vi "Get subnet.vi"() -> (14 "Subnet":string[](array[string]))   [LabVIEW 2026]
doc: "Calls system specific operating system function and returns subnet broadcast addresses of all installed network cards. Supports Windows (default case, calls IPCONFIG), Unix (calls IFCONFIG) and Mac.OS (calls IFCONFIG)."
panel:
  out "IP address":string[](array[string])
  out "Subnet mask":string[](array[string])
  out "Sum":i32[][](array[numeric])
  out "IPCONFIG Output":string
  # "Calls IPCONFIG and returns subnet broadcast addresses of all installed network cards."
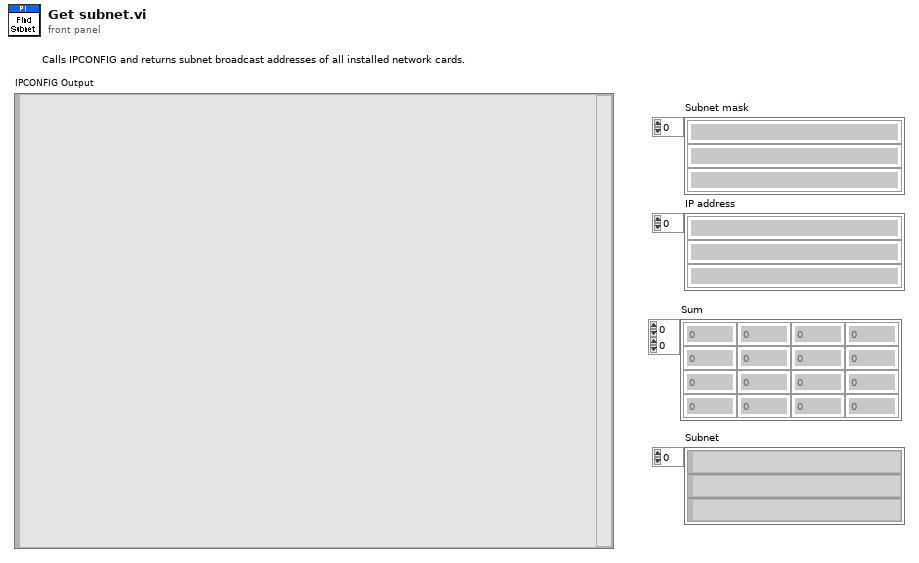
[diagram p1: front panel]
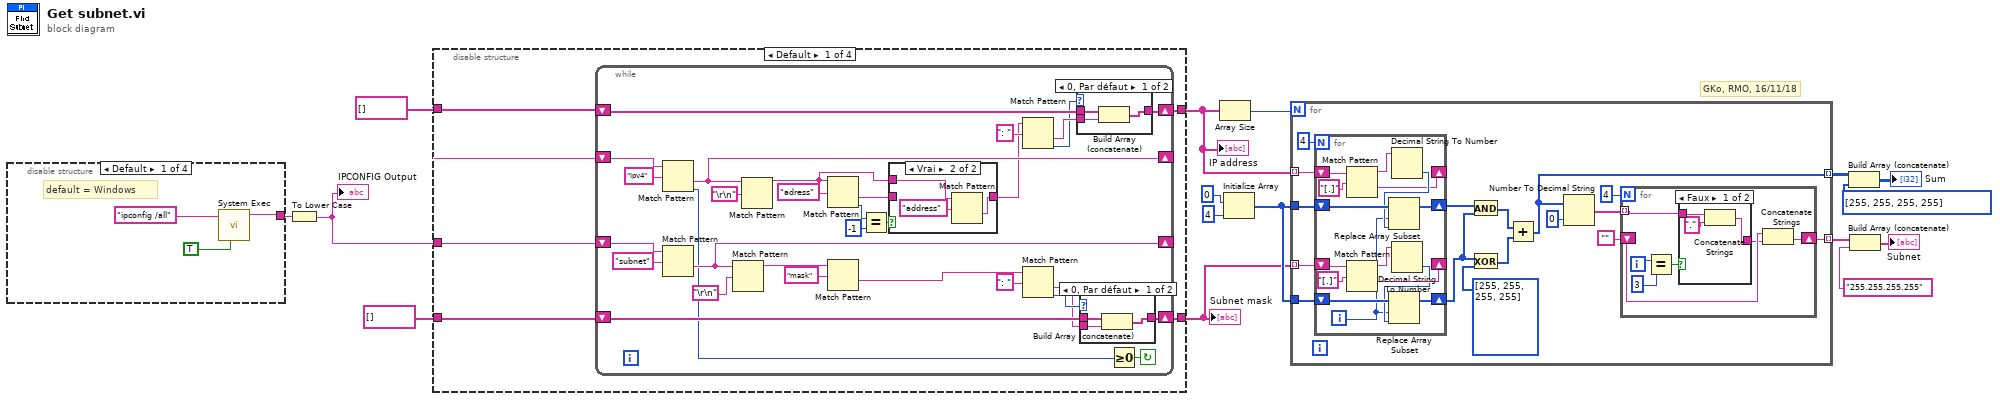
[diagram p0: block diagram]
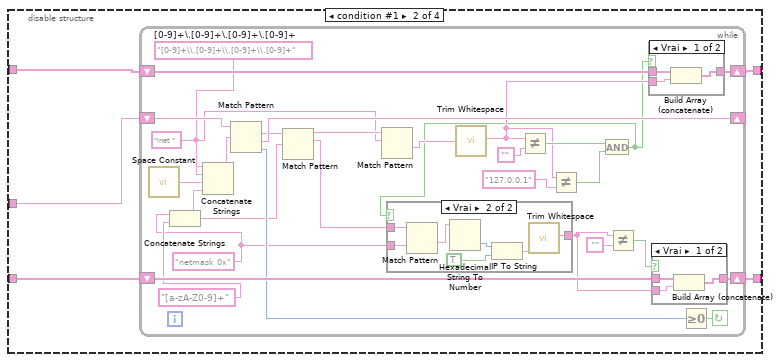
[diagram p5: hidden frame]
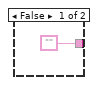
[diagram p6: hidden frame]
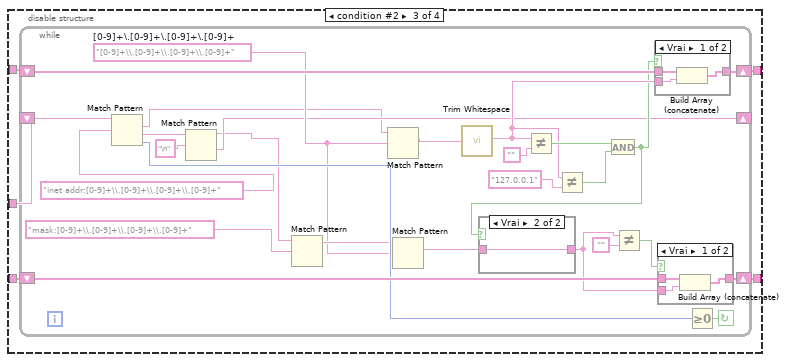
[diagram p9: hidden frame]
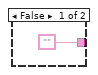
[diagram p10: hidden frame]
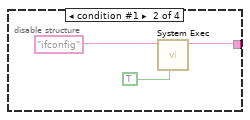
[diagram p14: hidden frame]
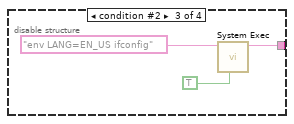
[diagram p15: hidden frame]
diagram:
  # "GKo, RMO, 16/11/18"
  n1 = disable-structure shown="Default" {
    disable-tunnel: [w17 w20 w23 _] -> w1
    frame condition #0 (active) {
      # "default = Windows"
      n2 = call <vilib>:"System Exec.vi"("run minimized? (F)"=TRUE, "command line"="ipconfig /all") -> ("standard output"=w17:string)  [unwired: 4 in, 5 out]
    }
    frame condition #1 {
      n3 = call <vilib>:"System Exec.vi"("run minimized? (F)"=TRUE, "command line"="ifconfig") -> ("standard output"=w20:string)  [unwired: 4 in, 5 out]
    }
    frame condition #2 {
      n4 = call <vilib>:"System Exec.vi"("run minimized? (F)"=TRUE, "command line"="env LANG=EN_US ifconfig") -> ("standard output"=w23:string)  [unwired: 4 in, 5 out]
    }
    frame condition #3 {
      # "No broadcasts on RT systems"
    }
  }
  n5 = To Lower Case(string=w1) -> (all lower case string=w15:string)
  "IPCONFIG Output" <- w15
  n6 = disable-structure shown="Default" {
    disable-tunnel: string[] [] -> [w30 w75 w125 w164]
    disable-tunnel: w15 -> [w29 w76 w124 _]
    disable-tunnel: string[] [] -> [w28 w77 w126 w165]
    disable-tunnel: [w27 w73 w122 w164] -> w9
    disable-tunnel: [w26 w74 w123 w165] -> w8
    frame condition #0 (active) {
      n7 = while {
        shift-right: [w55] -> _
        shift-left: w29 -> [w60]
        shift-right: [w52] -> w27
        shift-left: w30 -> [w53]
        shift-right: [w37] -> _
        shift-left: w29 -> [w43]
        shift-right: [w40] -> w26
        shift-left: w28 -> [w41]
        stop <- w56 continue-if-true
        n8 = Match Pattern(string=w43, regular expression="ipv4") -> (after substring=w37:string, offset past match=w38:i32)  [unwired: 3 out]
        n9 = Match Pattern(string=w60, regular expression="subnet") -> (after substring=w55:string)  [unwired: 4 out]
        n10 = Match Pattern(string=w55, regular expression="\r\n") -> (before substring=w49:string)  [unwired: 4 out]
        n11 = Match Pattern(string=w37, regular expression="\r\n") -> (before substring=w31:string)  [unwired: 4 out]
        n12 = Match Pattern(string=w31, regular expression="adress") -> (after substring=w33:string, offset past match=w36:i32)  [unwired: 3 out]
        n13 = Match Pattern(string=w49, regular expression="mask") -> (after substring=w48:string)  [unwired: 4 out]
        n14 = Equal?(x=w36, y=-1) -> (x = y?=w34:bool)
        n15 = case shown="Vrai" w34 {
          tunnel: w33 -> [w61 _]
          tunnel: [w61 w62] -> w32
          tunnel: w31 -> [_ w63]
          frame False {
          }
          frame True {
            n16 = Match Pattern(string=w63, regular expression="address") -> (after substring=w62:string)  [unwired: 4 out]
          }
        }
        n17 = Match Pattern(string=w32, regular expression=": ") -> (after substring=w42:string, offset past match=w39:i32)  [unwired: 3 out]
        n18 = Match Pattern(string=w48, regular expression=": ") -> (after substring=w51:string, offset past match=w54:i32)  [unwired: 3 out]
        n19 = case shown="0, Par défaut" w39 {
          tunnel: w41 -> [w67 w68]
          tunnel: [w65 w68] -> w40
          tunnel: w42 -> [w66 _]
          frame 0, Default {
            n20 = Build Array (concatenate)(w67, w66) -> (w65:string[])
          }
          frame -1 {
          }
        }
        n21 = case shown="0, Par défaut" w54 {
          tunnel: w53 -> [w71 w72]
          tunnel: [w69 w72] -> w52
          tunnel: w51 -> [w70 _]
          frame 0, Default {
            n22 = Build Array (concatenate)(w71, w70) -> (w69:string[])
          }
          frame -1 {
          }
        }
        n23 = Greater Or Equal To 0?(x=w38) -> (x >= 0?=w56:bool)
      }
    }
    frame condition #1 {
      n24 = while {
        shift-right: [w103] -> w73
        shift-left: w75 -> [w104]
        shift-right: [w98] -> _
        shift-left: w76 -> [w102]
        shift-right: [w100] -> w74
        shift-left: w77 -> [w101]
        stop <- w105 continue-if-true
        w85 = "[0-9]+\\.[0-9]+\\.[0-9]+\\.[0-9]+"  # [0-9]+\.[0-9]+\.[0-9]+\.[0-9]+
        w80 = "inet " ("regular expression")
        w89 = "netmask 0x" ("regular expression")
        n25 = call <vilib>:"Space Constant.vi"() -> ("String"=w84:string)
        n26 = Concatenate Strings(w89, "[a-zA-Z0-9]+") -> (w83:string)
        n27 = Concatenate Strings(w80, w85, w84, w83) -> (w86:string)
        n28 = Match Pattern(string=w102, regular expression=w86) -> (match substring=w82:string, after substring=w98:string, offset past match=w99:i32)  [unwired: 2 out]
        n29 = Match Pattern(string=w82, regular expression=w83) -> (before substring=w81:string, match substring=w88:string)  [unwired: 3 out]
        n30 = Match Pattern(string=w81, regular expression=w80) -> (after substring=w79:string)  [unwired: 4 out]
        n31 = call <vilib>:"Trim Whitespace.vi"("string"=w79) -> ("trimmed string"=w92:string)  [unwired: 1 in]
        n32 = Not Equal?(x=w92, y="") -> (x != y?=w93:bool)
        n33 = Not Equal?(x=w92, y="127.0.0.1") -> (x != y?=w87:bool)
        n34 = And(x=w93, y=w87) -> (x .and. y?=w78:bool)
        n35 = case shown="Vrai" w78 {
          tunnel: ["" w113] -> w95
          tunnel: w89 -> [_ w111]
          tunnel: w88 -> [_ w107]
          frame False {
          }
          frame True {
            n36 = Match Pattern(string=w107, regular expression=w111) -> (after substring=w112:string)  [unwired: 4 out]
            n37 = Hexadecimal String To Number(string=w112) -> (number=w110:u32)  [unwired: 3 out]
            n38 = IP To String(1:TRUE, 2:w110) -> (0:w109:string)
            n39 = call <vilib>:"Trim Whitespace.vi"("string"=w109) -> ("trimmed string"=w113:string)  [unwired: 1 in]
          }
        }
        n40 = Not Equal?(x=w95, y="") -> (x != y?=w94:bool)
        n41 = case shown="Vrai" w78 {
          tunnel: w101 -> [w116 w117]
          tunnel: [w115 w117] -> w100
          tunnel: w92 -> [w114 _]
          frame True {
            n42 = Build Array (concatenate)(w116, w114) -> (w115:string[])
          }
          frame False {
          }
        }
        n43 = case shown="Vrai" w94 {
          tunnel: w104 -> [w120 w121]
          tunnel: [w119 w121] -> w103
          tunnel: w95 -> [w118 _]
          frame True {
            n44 = Build Array (concatenate)(w120, w118) -> (w119:string[])
          }
          frame False {
          }
        }
        n45 = Greater Or Equal To 0?(x=w99) -> (x >= 0?=w105:bool)
      }
    }
    frame condition #2 {
      n46 = while {
        shift-right: [w151] -> w122
        shift-left: w125 -> [w152]
        shift-right: [w131] -> _
        shift-left: w124 -> [w150]
        shift-right: [w148] -> w123
        shift-left: w126 -> [w149]
        stop <- w153 continue-if-true
        w137 = "[0-9]+\\.[0-9]+\\.[0-9]+\\.[0-9]+"  # [0-9]+\.[0-9]+\.[0-9]+\.[0-9]+
        n47 = Match Pattern(string=w150, regular expression="inet addr:[0-9]+\\.[0-9]+\\.[0-9]+\\.[0-9]+") -> (match substring=w127:string, after substring=w130:string, offset past match=w147:i32)  [unwired: 2 out]
        n48 = Match Pattern(string=w130, regular expression="\n") -> (before substring=w128:string, after substring=w131:string)  [unwired: 3 out]
        n49 = Match Pattern(string=w128, regular expression="mask:[0-9]+\\.[0-9]+\\.[0-9]+\\.[0-9]+") -> (match substring=w138:string)  [unwired: 4 out]
        n50 = Match Pattern(string=w127, regular expression=w137) -> (match substring=w140:string)  [unwired: 4 out]
        n51 = Match Pattern(string=w138, regular expression=w137) -> (match substring=w136:string)  [unwired: 4 out]
        n52 = call <vilib>:"Trim Whitespace.vi"("string"=w140) -> ("trimmed string"=w142:string)  [unwired: 1 in]
        n53 = Not Equal?(x=w142, y="") -> (x != y?=w143:bool)
        n54 = Not Equal?(x=w142, y="127.0.0.1") -> (x != y?=w133:bool)
        n55 = And(x=w143, y=w133) -> (x .and. y?=w134:bool)
        n56 = case shown="Vrai" w134 {
          tunnel: w136 -> [_ w155]
          tunnel: ["" w155] -> w135
          frame False {
          }
          frame True {
          }
        }
        n57 = Not Equal?(x=w135, y="") -> (x != y?=w144:bool)
        n58 = case shown="Vrai" w134 {
          tunnel: w149 -> [w158 w159]
          tunnel: [w157 w159] -> w148
          tunnel: w142 -> [w156 _]
          frame True {
            n59 = Build Array (concatenate)(w158, w156) -> (w157:string[])
          }
          frame False {
          }
        }
        n60 = case shown="Vrai" w144 {
          tunnel: w152 -> [w162 w163]
          tunnel: [w161 w163] -> w151
          tunnel: w135 -> [w160 _]
          frame True {
            n61 = Build Array (concatenate)(w162, w160) -> (w161:string[])
          }
          frame False {
          }
        }
        n62 = Greater Or Equal To 0?(x=w147) -> (x >= 0?=w153:bool)
      }
    }
    frame condition #3 {
      # "No broadcasts on RT systems"
    }
  }
  "Subnet mask" <- w9
  "IP address" <- w8
  n63 = Array Size(array=w8) -> (size(s)=w13:i32)
  n64 = Initialize Array(0, 4 ("dimension size")) -> (w10:i32[])
  n65 = for {
    N: w13 -> [_]
    tunnel: w8 -> [w180] mode=indexing
    tunnel: w10 -> [w179]
    tunnel: w9 -> [w178] mode=indexing
    tunnel: w10 -> [w177]
    tunnel: [w167] -> w7 mode=indexing
    tunnel: [w166] -> w4 mode=indexing
    n66 = for {
      N: 4 -> [_]
      shift-right: [w202] -> _
      shift-left: w180 -> [w207]
      shift-right: [w201] -> w169
      shift-left: w179 -> [w205]
      shift-right: [w197] -> w168
      shift-left: w177 -> [w198]
      shift-right: [w195] -> _
      shift-left: w178 -> [w196]
      i -> [w193]
      n67 = Match Pattern(string=w207, regular expression="[.]") -> (before substring=w204:string, after substring=w202:string)  [unwired: 3 out]
      n68 = Match Pattern(string=w196, regular expression="[.]") -> (before substring=w199:string, after substring=w195:string)  [unwired: 3 out]
      n69 = Decimal String To Number(string=w204) -> (number=w203:i32)  [unwired: 3 out]
      n70 = Replace Array Subset(array=w205, new element=w203, index=w193) -> (w201:i32[])
      n71 = Decimal String To Number(string=w199) -> (number=w194:i32)  [unwired: 3 out]
      n72 = Replace Array Subset(array=w198, new element=w194, index=w193) -> (w197:i32[])
    }
    n73 = And(x=w169, y=w168) -> (x .and. y?=w171:i32[])
    n74 = Exclusive Or(1:i32[] [255, 255, 255, 255], 2:w168) -> (0:w172:i32[])
    n75 = Add(x=w171, y=w172) -> (x+y=w166:i32[])
    n76 = Number To Decimal String(number=w166, width (-)=i16 0) -> (decimal integer string=w175:string[])
    n77 = for {
      N: 4 -> [_]
      tunnel: w175 -> [w185] mode=indexing
      shift-right: [w184] -> w167
      shift-left: "" -> [w183]
      i -> [w188]
      n78 = Equal?(x=w188, y=3) -> (x = y?=w186:bool)
      n79 = case shown="Faux" w186 {
        tunnel: w185 -> [w190 w192]
        tunnel: [w189 w192] -> w182
        frame False {
          n80 = Concatenate Strings(w190, "." ("string")) -> (w189:string)
        }
        frame True {
        }
      }
      n81 = Concatenate Strings(w183, w182) -> (w184:string)
    }
  }
  n82 = Build Array (concatenate)(w4, i32[] [255, 255, 255, 255] ("x+y")) -> (→"Sum":i32[][])
  n83 = Build Array (concatenate)(w7, "255.255.255.255") -> (→"Subnet":string[])
